vi "Stop Acquisition.vi"(8 "error in (no error)":errorcluster, 11 "Acquisition Configuration in":T1) -> (0 "error out":errorcluster)   [LabVIEW 2020, in "ChromTech Next Gen Compensator Pump.lvlib" / "Acquisition.lvlib"]
doc: "Stops the acquisition."
uses:
  Acquisition.lvlib
  Hardware Configuration.ctl
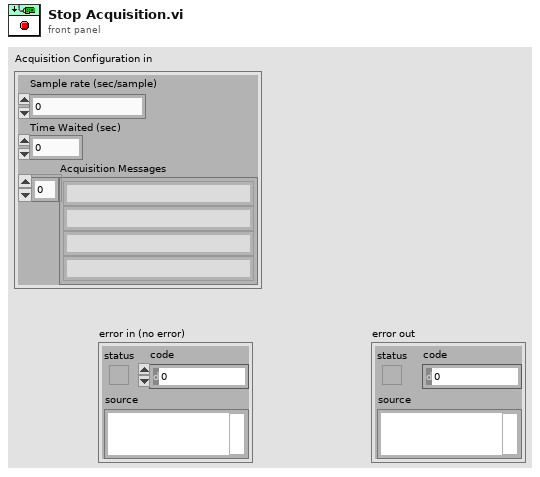
[diagram p1: front panel]
types:
  T1 = typedef "ChromTech Next Gen Compensator Pump.lvlib/Acquisition.lvlib/Hardware Configuration.ctl" = cluster{"Sample rate (sec/sample)":dbl, "Time Waited (sec)":dbl, "Acquisition Messages":string[]}
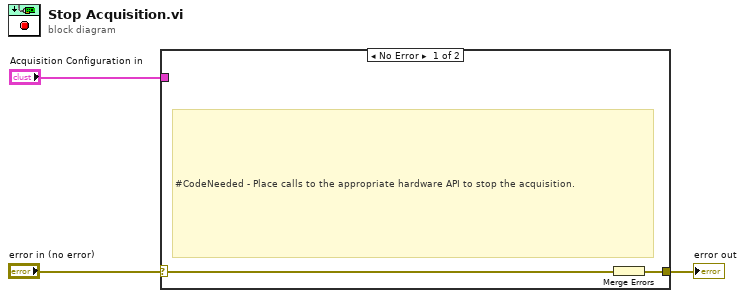
[diagram p0: block diagram]
diagram:
  n1 = case shown="No Error" "error in (no error)" {
    selector: "error in (no error)" -> [w4 w6]
    tunnel: [w5 w6] -> w2
    tunnel: "Acquisition Configuration in" -> [_ _]
    frame No Error {
      # "#CodeNeeded - Place calls to the appropriate hardware API to stop the acquisition."
      n2 = Merge Errors(w4) -> (w5:errorcluster)
    }
    frame Error {
    }
  }
  "error out" <- w2
